vi "Send OCP.vi"(8 "error in":errorcluster, 11 "6700C in":refnum<class "6700C.lvclass">) -> (0 "error out":errorcluster, 3 "6700C out":refnum<class "6700C.lvclass">)   [LabVIEW 2019, in "6700C.lvlib" / "6700C.lvclass"]
uses:
  Library/6700C.lvclass
  C:/Users/Public/Documents/Development/builds/Instruments/PowerSupply.lvlibp/Library/PowerSupply.lvclass
  Library/6700C.lvclass/6700C.ctl
  Accessors/Write Local Resource.vi
  Accessors/Read Local Resource.vi
  builds/Instruments/PowerSupply.lvlibp/Accessors/Read Active Channel.vi
  <instrlib>/Agilent N6700 Series/Agilent N6700 Series.lvlib
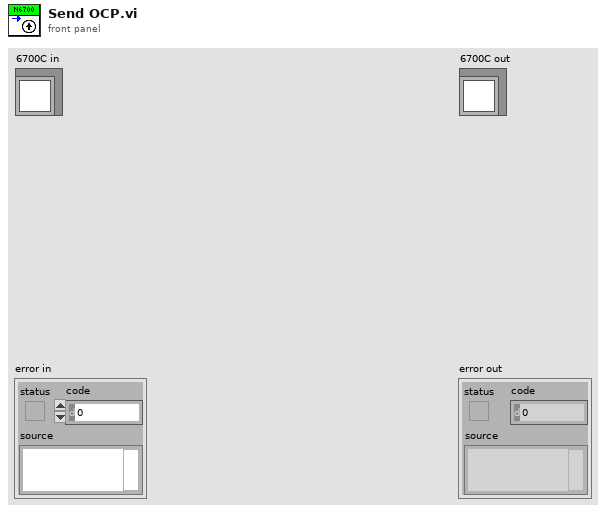
[diagram p1: front panel]
types:
  T1 = typedef "PowerSupply.lvlibp/PowerSupply.lvclass/OCP Mode.ctl" = enum16{"Shutdown", "Foldback"}
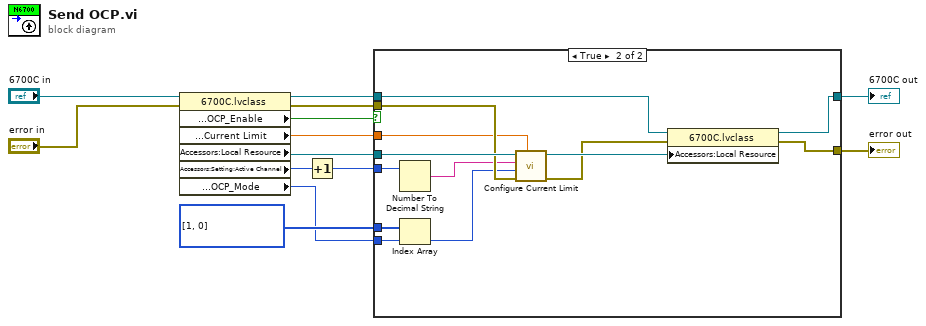
[diagram p0: block diagram]
diagram:
  w4 = i32[] [1, 0] items=["Regulatory Limit", "Trip Limit"]
  n1 = property class="6700C.lvclass"(reference="6700C in", error in="error in") -> (reference out=w7:refnum<class "6700C.lvclass">, error out=w8:errorcluster, "Accessors:Setting:Protection:OCP_Enable"=w1:bool, "Accessors:Setting:Protection:Current Limit"=w6:dbl, "Accessors:Local Resource"=w9:refnum<visa-resource-name>, "Accessors:Setting:Active Channel"=w5:u32, "Accessors:Setting:Protection:OCP_Mode"=w3:T1)
  n2 = Increment(x=w5) -> (x+1=w2:u32)
  n3 = case shown="True" w1 {
    tunnel: [w14 w28] -> w13
    tunnel: [w15 w27] -> w12
    tunnel: w9 -> [_ w26]
    tunnel: w8 -> [w14 w25]
    tunnel: w7 -> [w15 w23]
    tunnel: w6 -> [_ w21]
    tunnel: w4 -> [_ w19]
    tunnel: w3 -> [_ w18]
    tunnel: w2 -> [_ w16]
    frame False {
    }
    frame True {
      n4 = Number To Decimal String(number=w16) -> (decimal integer string=w20:string)  [unwired: 1 in]
      n5 = Index Array(array=w19, index=w18) -> (element=w17:i32)
      n6 = call <instrlib>:"Configure Current Limit.vi"("Limit (0.0 amps)"=w21, "error in (no error)"=w25, "Behavior (0: Regulatory Limit)"=w17, "Channel Name (1)"=w20, "VISA resource name"=w26) -> ("error out"=w22:errorcluster, "VISA resource name out"=w24:refnum<visa-resource-name>)  [unwired: 5 in]
      n7 = property class="6700C.lvclass"(reference=w23, error in=w22, "Accessors:Local Resource"=w24) -> (reference out=w27:refnum<class "6700C.lvclass">, error out=w28:errorcluster)
    }
  }
  "error out" <- w13
  "6700C out" <- w12
